vi "CRYFrequency Show.vi"(8 "Frequency Splitter Position":dbl, 10 "FrequencyShow":bool, 11 "pGraph VI":refnum<vi>) -> ()   [LabVIEW 2013]
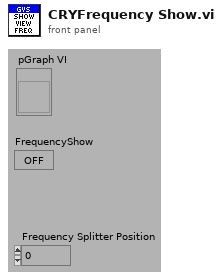
[diagram p1: front panel]
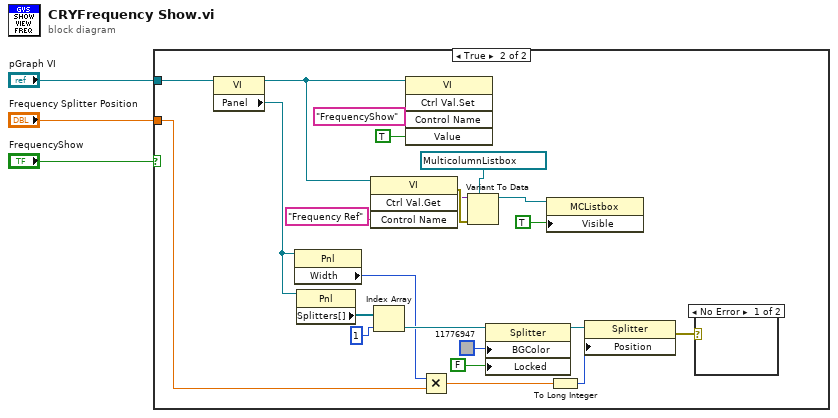
[diagram p0: block diagram]
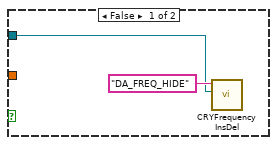
[diagram p2: hidden frame]
diagram:
  n1 = case shown="True" "FrequencyShow" {
    tunnel: "Frequency Splitter Position" -> [_ w27]
    tunnel: "pGraph VI" -> [w4 w7]
    frame False {
      n2 = call "CRYFrequency InsDel.vi"("Graph VI Ref"=w4, "sAction"="DA_FREQ_HIDE") -> ()  [unwired: 10 in]
    }
    frame True {
      n3 = property class="VI"(reference=w7) -> (reference out=w26:refnum<vi>, "Panel"=w25:refnum<vi>)  [unwired: 1 in, 1 out]
      n4 = property class="Pnl"(reference=w25) -> ("Width"=w10:u32)  [unwired: 1 in, 2 out]
      n5 = property class="Pnl"(reference=w25) -> ("Splitters[]"=w16:refnum<vi>[])  [unwired: 1 in, 2 out]
      n6 = invoke class="VI" method="Ctrl Val.Get"(reference=w26, "Control Name"="Frequency Ref") -> (error out=w22:errorcluster, "Get Control Value Variant"=w21:variant)  [unwired: 2 in, 2 out]
      n7 = Index Array(array=w16, index=1) -> (element=w14:refnum<vi>)
      n8 = invoke class="VI" method="Ctrl Val.Set"(reference=w26, "Control Name"="FrequencyShow", "Value"=TRUE ("Visible")) -> ()  [unwired: 2 in, 5 out]
      n9 = Multiply(x=w10, y=w27) -> (x*y=w9:dbl)
      n10 = Variant To Data(error in=w22, type=refnum<vi> refnum ("Legend Ref"), Variant=w21) -> (data=w17:refnum<vi>)  [unwired: 1 out]
      n11 = property on="Property Node" class="Splitter"(reference=w14, "BGColor"=u32 11776947, "Locked"=FALSE ("Splitter Position Locked")) -> (reference out=w11:refnum<vi>)  [unwired: 1 in, 1 out]
      n12 = property class="MCListbox"(reference=w17, "Visible"=TRUE) -> ()  [unwired: 1 in, 2 out]
      n13 = To Long Integer(number=w9) -> (32bit integer=w8:i32)
      n14 = property on="Property Node" class="Splitter"(reference=w11, "Position"=w8) -> (error out=w6:errorcluster)  [unwired: 1 in, 1 out]
      n15 = case shown="No Error" w6 {
        frame No Error {
        }
        frame Error {
        }
      }
    }
  }
